vi "calcForceError.vi"(8 "error in (no error)":errorcluster, 11 "Model in":refnum<class "Model.lvclass">) -> (0 "error out":errorcluster, 3 "Model out":refnum<class "Model.lvclass">)   [LabVIEW 2013, in "Model.lvclass"]
uses:
  Model.lvclass
  Typedefs/ControllerData.ctl
  Typedefs/ForceDemand.ctl
  Model.lvclass/Model.ctl
  ApplicationElements/ForceSensor/ForceSensor.lvclass/ForceSensor.ctl
  ApplicationElements/Logger/Logger.lvclass/Logger.ctl
  ApplicationElements/SystemController/SystemController.lvclass
  ApplicationElements/ForceSensor/ForceSensor.lvclass
  Typedefs/M2AADTTypedefs.lvlib
  ApplicationElements/Logger/Logger.lvclass
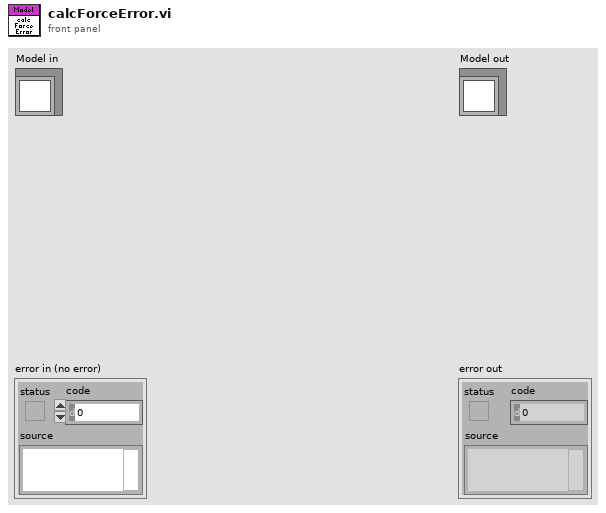
[diagram p1: front panel]
types:
  T1 = typedef "M2AADTTypedefs.lvlib/ControllerData.ctl" = cluster{"Force Demand":T2, "Force Error":T2}
  T2 = typedef "M2AADTTypedefs.lvlib/ForceDemand.ctl" = dbl[unit]
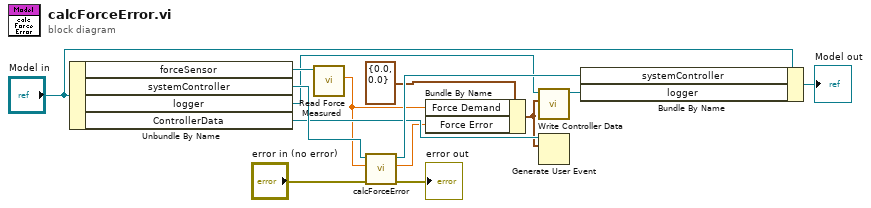
[diagram p0: block diagram]
diagram:
  n1 = Unbundle By Name("Model in") -> ("forceSensor"=w10:refnum<class "ForceSensor.lvclass">, "systemController"=w14:refnum<class "SystemController.lvclass">, "logger"=w3:refnum<class "Logger.lvclass">, "ControllerData"=w7:refnum<user-event>)
  n2 = call "Read Force Measured.vi"("ForceSensor in"=w10) -> ("Force Demand"=w5:T2)  [unwired: 9 in, 1 out]
  n3 = call "calcForceError.vi"("error in (no error)"="error in (no error)", "Force Measured"=w5, "SystemController in"=w14) -> ("error out"=→"error out":errorcluster, "Force Error"=w4:T2, "SystemController out"=w11:refnum<class "SystemController.lvclass">)  [unwired: 6 in]
  n4 = Bundle By Name(cluster=T1 {"Force Demand"=0.0, "Force Error"=0.0} ("event data"), "Force Demand"=w5, "Force Error"=w4) -> (w1:T1)
  n5 = call "Write Controller Data.vi"("Controller Data"=w1, "Logger in"=w3) -> ("Logger out"=w2:refnum<class "Logger.lvclass">)  [unwired: 9 in]
  n6 = Generate User Event(user event=w7, event data cluster=w1) -> ()  [unwired: 2 in, 2 out]
  n7 = Bundle By Name(cluster="Model in", "systemController"=w11, "logger"=w2) -> (→"Model out":refnum<class "Model.lvclass">)
